vi "Agilent 34401 Read Multiple Measurements.vi"() -> ()   [LabVIEW 2021]
doc: "This example shows how to configure a measurement and take multiple readings."
uses:
  <instrlib>/Agilent 34401/Public/Data/Read (Multiple Points).vi
  <instrlib>/Agilent 34401/Agilent 34401.lvlib
panel:
  out "error out":errorcluster
  in  "error in":errorcluster
  in  "Function":u16(ring) items=["DC Voltage", "AC Voltage", "2 - Wire Resistance", "4 - Wire Resistance", "DC Current", "AC Current", "Frequency", "Period", "Continuity", "Diode Checking", "VDC:VDC Ratio", "Temperature", "Capacitance"]
  in  "Maximum Time":u32=10000
  in  "Sample Count":i32=10
  out "Measurements":dbl[](array[numeric])
  in  "Agilent Fgen":refnum<visa-resource-name> caption="VISA resource name"
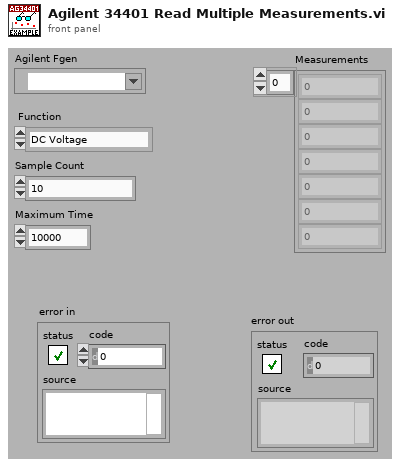
[diagram p1: front panel]
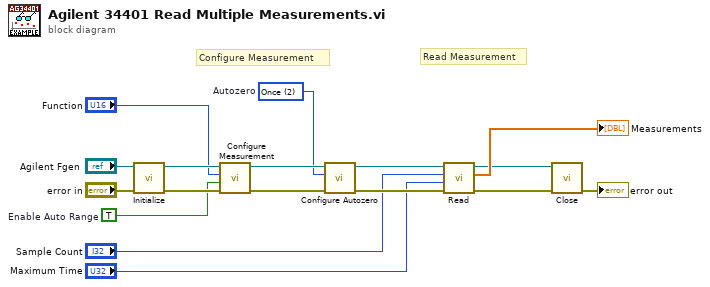
[diagram p0: block diagram]
diagram:
  w10 = u16 2 items=["On", "Off", "Once"]  # Autozero
  w14 = TRUE  # Enable Auto Range
  # "Read Measurement"
  # "Configure Measurement"
  n1 = call <instrlib>:"Initialize.vi"("error in (no error)"="error in", "VISA resource name"="Agilent Fgen") -> ("error out"=w15:errorcluster, "VISA resource name out"=w16:refnum<visa-resource-name>)  [unwired: 8 in]
  n2 = call <instrlib>:"Configure Measurement.vi"("error in (no error)"=w15, "Enable Auto Range (T: Enable)"=w14, "Function (0: DC Voltage)"="Function", "VISA resource name"=w16) -> ("error out"=w12:errorcluster, "VISA resource name out"=w11:refnum<visa-resource-name>)  [unwired: 6 in]
  n3 = call <instrlib>:"Configure Autozero.vi"("error in (no error)"=w12, "Autozero  (0: On)"=w10, "VISA resource name"=w11) -> ("error out"=w6:errorcluster, "VISA resource name out"=w7:refnum<visa-resource-name>)  [unwired: 7 in]
  n4 = call-poly <instrlib>:"Read.vi"("error in (no error)"=w6, "Maximum Time (10000 ms)"="Maximum Time", "Sample Count (1)"="Sample Count", "VISA resource name"=w7) -> ("error out"=w8:errorcluster, "Measurements"=→"Measurements":dbl[], "VISA resource name out"=w9:refnum<visa-resource-name>)  [unwired: 5 in]
  n5 = call <instrlib>:"Close.vi"("error in (no error)"=w8, "VISA resource name"=w9) -> ("error out"=→"error out":errorcluster)  [unwired: 9 in]
